vi "module-05-sample-5-1.vi"() -> ()   [LabVIEW 2019]
uses:
  <vilib>/Rock Robotics/WPI/ThirdParty/JAS_Junk/TrajLib/Timer_New.vi
  <vilib>/Rock Robotics/WPI/ThirdParty/JAS_Junk/TrajLib/Timer_Start.vi
  <vilib>/Rock Robotics/WPI/ThirdParty/JAS_Junk/TrajLib/Timer_HasPeriodPassedOnce.vi
  samples-common-library/Ctrl_Training_Library_Protected/CtrlTrainingLibary_Protected.lvlib
  <vilib>/Rock Robotics/WPI/ThirdParty/JAS_Junk/TrajLib/Trajectory_Library.lvlib
panel:
  in  "Tab Control":enum32{"Execution", "Logic"}(tab)
  in  "Driver Gather Cube":bool
  in  "Driver Cancel Button":bool
  out "Request GO":bool
  out "Digital State Chart":cluster{dbl, dbl, dbl, dbl, dbl, dbl}(graph)
  out "Ready":bool
  out "Arm Extend Cmd":bool
  out "Hand Close Cmd":bool
  out "Cur Time":dbl format="%20.3f"
  # "Training Sample 5.1\nSequential Logic"
  # "F1"
  # "F2"
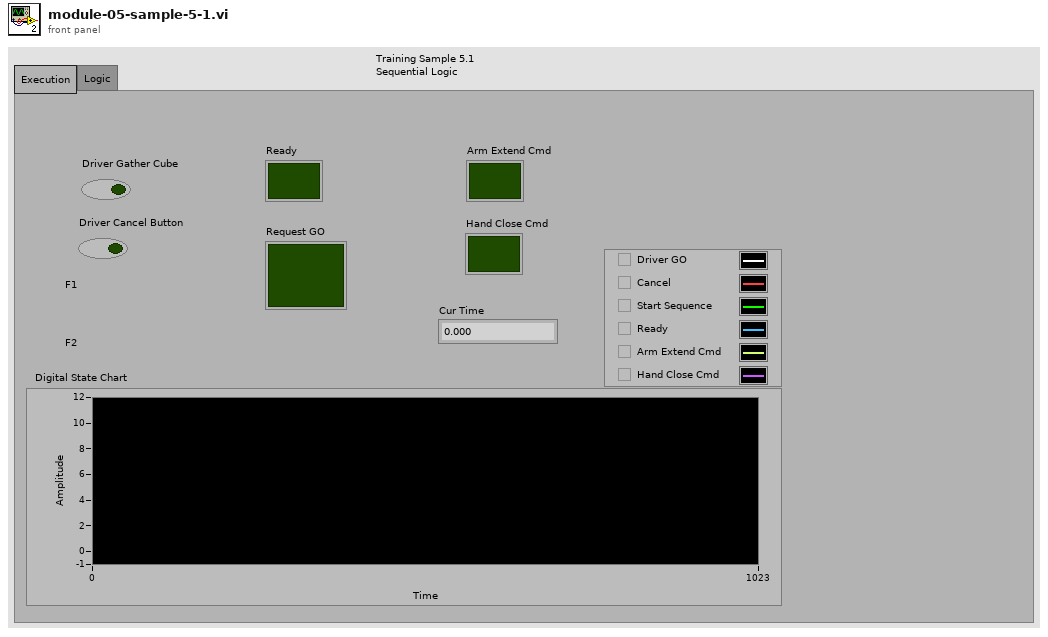
[diagram p1: front panel]
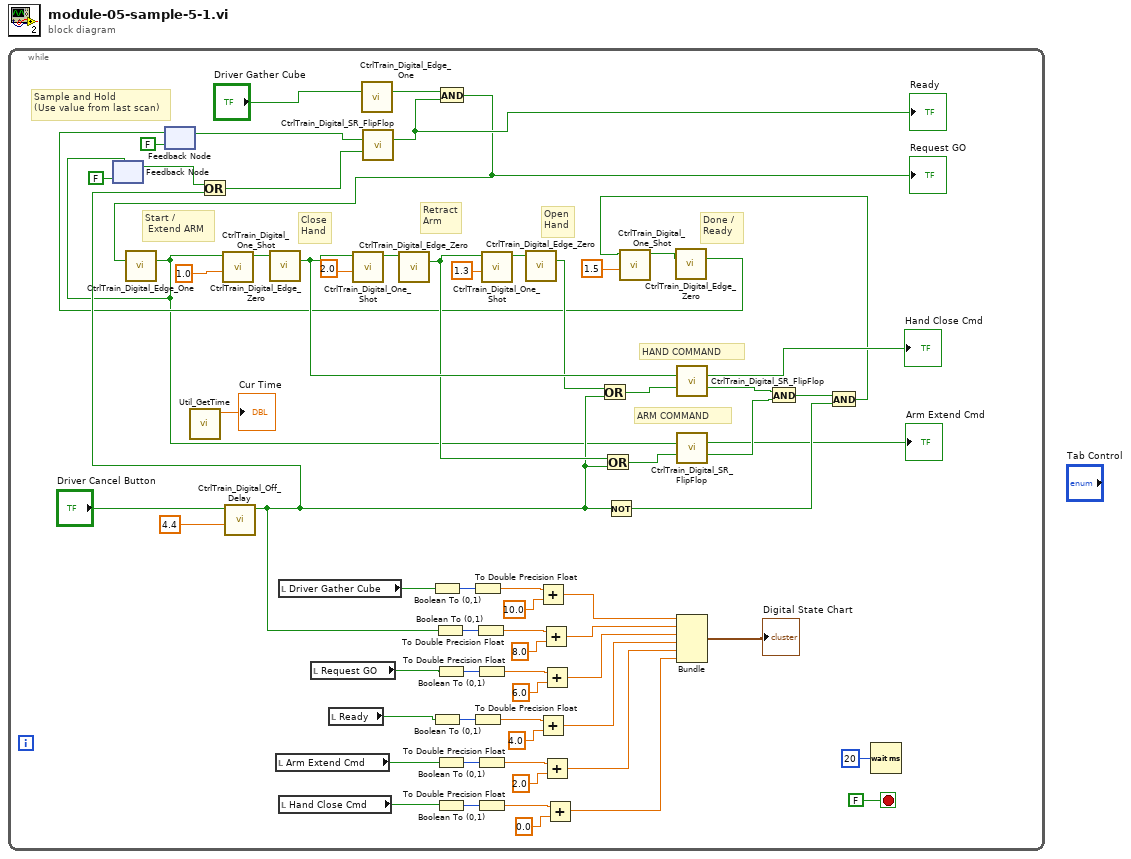
[diagram p0: block diagram]
diagram:
  n1 = while {
    stop <- FALSE stop-if-true
    # "Sample and Hold\n(Use value from last scan)"
    # "Done / \nReady"
    # "Open\nHand"
    # "Retract\nArm"
    # "Close\nHand"
    # "Start /\n Extend ARM"
    # "HAND COMMAND"
    # "ARM COMMAND"
    n2 = feedback #1(FALSE ("Arm Extend Cmd")) -> (w3:bool)
    n3 = feedback #2(FALSE ("Arm Extend Cmd")) -> (w7:bool)
    n4 = call <vilib>:"Util_GetTime.vi"() -> ("FPGA_Time_Seconds"=→"Cur Time":dbl)  [unwired: 10 in, 1 out]
    n5 = call "CtrlTrain_Digital_Off_Delay.vi"("Delay"=4.4 ("OneShot"), "Input"="Driver Cancel Button") -> ("Output"=w10:bool)  [unwired: 8 in, 1 out]
    n6 = Or(x=w3, y=w10) -> (x .or. y?=w13:bool)
    n7 = local read "Arm Extend Cmd"() -> (w17:bool)
    n8 = local read "Driver Gather Cube"() -> (w21:bool)
    n9 = local read "Hand Close Cmd"() -> (w18:bool)
    n10 = local read "Request GO"() -> (w15:bool)
    n11 = local read "Ready"() -> (w14:bool)
    n12 = call "CtrlTrain_Digital_Edge_One.vi"("Input"="Driver Gather Cube") -> ("Output"=w11:bool)  [unwired: 14 in]
    n13 = call "CtrlTrain_Digital_SR_FlipFlop.vi"("Set"=w7, "Reset"=w13) -> ("Output"=w16:bool)  [unwired: 12 in, 1 out]
    "Ready" <- w16
    n14 = Boolean To (0,1)(Boolean=w21) -> (0, 1=w65:i16)
    n15 = Boolean To (0,1)(Boolean=w14) -> (0, 1=w63:i16)
    n16 = Boolean To (0,1)(Boolean=w10) -> (0, 1=w60:i16)
    n17 = Boolean To (0,1)(Boolean=w15) -> (0, 1=w57:i16)
    n18 = Boolean To (0,1)(Boolean=w17) -> (0, 1=w54:i16)
    n19 = Boolean To (0,1)(Boolean=w18) -> (0, 1=w51:i16)
    n20 = And(x=w11, y=w16) -> (x .and. y?=w9:bool)
    "Request GO" <- w9
    n21 = call "CtrlTrain_Digital_Edge_One.vi"("Input"=w9) -> ("Output"=w2:bool)  [unwired: 14 in]
    n22 = feedback-in #1(w2) -> ()
    n23 = call "CtrlTrain_Digital_One_Shot.vi"("OneShot"=1.0, "Input"=w2) -> ("Output"=w39:bool)  [unwired: 8 in, 1 out]
    n24 = call "CtrlTrain_Digital_Edge_Zero.vi"("Input"=w39) -> ("Output"=w30:bool)  [unwired: 14 in]
    n25 = call "CtrlTrain_Digital_One_Shot.vi"("OneShot"=2.0, "Input"=w30) -> ("Output"=w38:bool)  [unwired: 8 in, 1 out]
    n26 = call "CtrlTrain_Digital_Edge_Zero.vi"("Input"=w38) -> ("Output"=w24:bool)  [unwired: 14 in]
    n27 = To Double Precision Float(number=w65) -> (double precision float=w42:dbl)
    n28 = To Double Precision Float(number=w63) -> (double precision float=w62:dbl)
    n29 = To Double Precision Float(number=w60) -> (double precision float=w59:dbl)
    n30 = To Double Precision Float(number=w57) -> (double precision float=w56:dbl)
    n31 = To Double Precision Float(number=w54) -> (double precision float=w53:dbl)
    n32 = To Double Precision Float(number=w51) -> (double precision float=w50:dbl)
    n33 = call "CtrlTrain_Digital_One_Shot.vi"("OneShot"=1.3, "Input"=w24) -> ("Output"=w37:bool)  [unwired: 8 in, 1 out]
    n34 = call "CtrlTrain_Digital_Edge_Zero.vi"("Input"=w37) -> ("Output"=w26:bool)  [unwired: 14 in]
    n35 = Add(x=w42, y=10.0) -> (x+y=w41:dbl)
    n36 = Add(x=w62, y=4.0) -> (x+y=w45:dbl)
    n37 = Add(x=w59, y=8.0) -> (x+y=w47:dbl)
    n38 = Add(x=w56, y=6.0) -> (x+y=w46:dbl)
    n39 = Add(x=w53, y=2.0) -> (x+y=w49:dbl)
    n40 = Add(x=w50, y=0.0) -> (x+y=w48:dbl)
    n41 = Or(x=w26, y=w10) -> (x .or. y?=w27:bool)
    n42 = Or(x=w24, y=w10) -> (x .or. y?=w25:bool)
    n43 = Not(x=w10) -> (.not. x?=w22:bool)
    n44 = call "CtrlTrain_Digital_SR_FlipFlop.vi"("Set"=w30, "Reset"=w27) -> ("Output"=→"Hand Close Cmd":bool, "Inverse Output"=w31:bool)  [unwired: 12 in]
    n45 = call "CtrlTrain_Digital_SR_FlipFlop.vi"("Set"=w2, "Reset"=w25) -> ("Output"=→"Arm Extend Cmd":bool, "Inverse Output"=w32:bool)  [unwired: 12 in]
    n46 = Bundle(w41, w47, w46, w45, w49, w48) -> (→"Digital State Chart":cluster{dbl, dbl, dbl, dbl, dbl, dbl})  [unwired: 1 in]
    n47 = And(x=w31, y=w32) -> (x .and. y?=w23:bool)
    n48 = And(x=w23, y=w22) -> (x .and. y?=w8:bool)
    n49 = call "CtrlTrain_Digital_One_Shot.vi"("OneShot"=1.5, "Input"=w8) -> ("Output"=w36:bool)  [unwired: 8 in, 1 out]
    n50 = call "CtrlTrain_Digital_Edge_Zero.vi"("Input"=w36) -> ("Output"=w5:bool)  [unwired: 14 in]
    n51 = feedback-in #2(w5) -> ()
    n52 = Wait (ms)(milliseconds to wait=u32 20) -> ()  [unwired: 1 out]
  }
